vi "Edit Triton.vi"(8 "error in":errorcluster, 11 "Instrument parameters in":T1) -> (0 "error out":errorcluster, 3 "Instrument parameters (out)":T1)   [LabVIEW 2025]
uses:
  MyTriton.lvlib
panel:
  in  "Max Trial Number":i32
  in  "Select channel":u16(ring)=8 items=["PT2 Head"=1, "PT2 Plate"=2, "Still Plate"=3, "Cold Plate"=4, "MC Plate Cernox"=5, "PT1 Head"=6, "PT1 Plate"=7, "MC Plate RuO2"=8, "Magnet"=13]
  in  "Auto clear error?":bool=TRUE
  in  "Hold at end?":bool=TRUE
  in  "Initialize magnet?":bool
  in  "Precision":dbl=0.001
  in  "stop":bool
  # "Settings for Triton..."
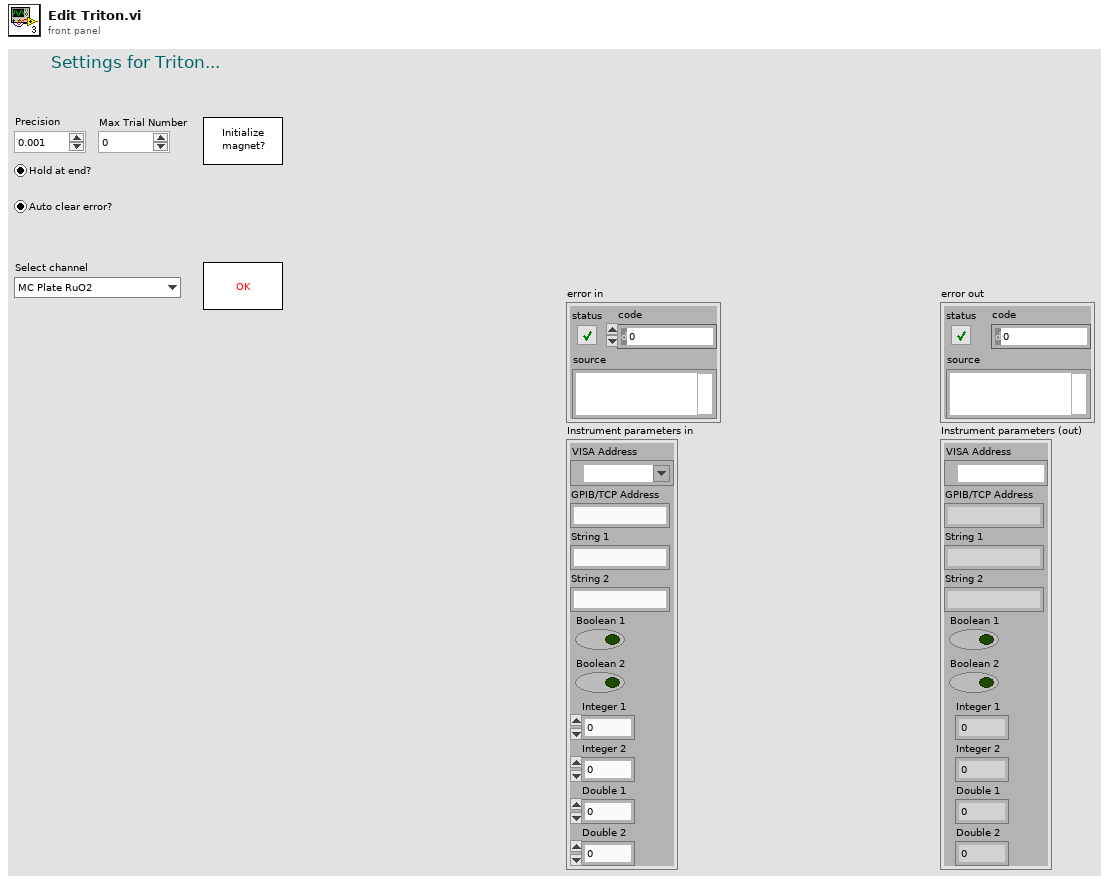
[diagram p1: front panel]
types:
  T1 = cluster{"VISA Address":refnum<visa-resource-name>, "GPIB/TCP Address":string, "String 1":string, "String 2":string, "Boolean 1":bool, "Boolean 2":bool, "Integer 1":i32, "Integer 2":i32, "Double 1":dbl, "Double 2":dbl}
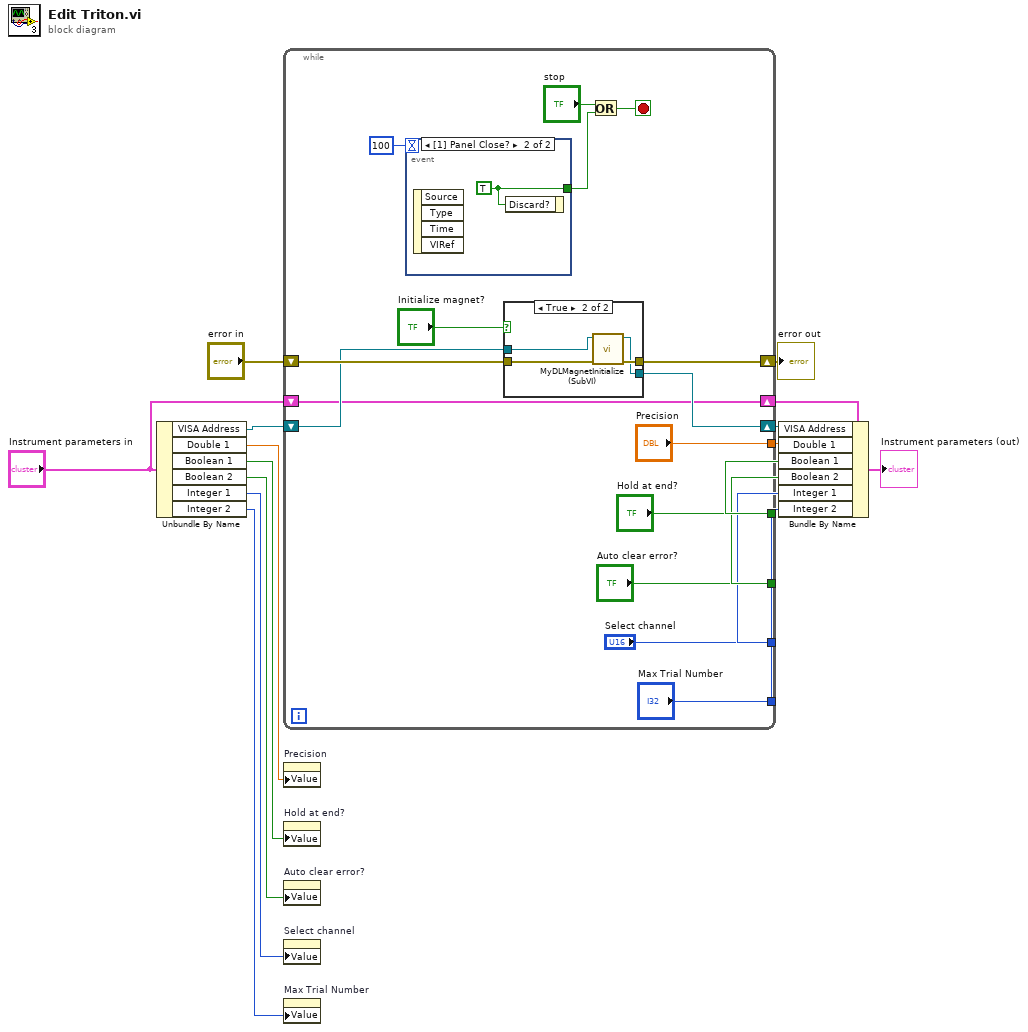
[diagram p0: block diagram]
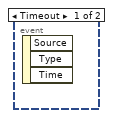
[diagram p3: hidden frame]
diagram:
  n1 = Unbundle By Name("Instrument parameters in") -> ("VISA Address"=w13:refnum<visa-resource-name>, "Double 1"=w14:dbl, "Boolean 1"=w5:bool, "Boolean 2"=w4:bool, "Integer 1"=w3:i32, "Integer 2"=w1:i32)
  n2 = while {
    shift-right: [w26] -> w16
    shift-left: "error in" -> [w27]
    shift-right: [w23] -> w11
    shift-left: "Instrument parameters in" -> [w23]
    shift-right: [w24] -> w10
    shift-left: w13 -> [w25]
    tunnel: ["Precision"] -> w12
    tunnel: ["Hold at end?"] -> w8
    tunnel: ["Auto clear error?"] -> w7
    tunnel: ["Select channel"] -> w6
    tunnel: ["Max Trial Number"] -> w2
    stop <- w29 stop-if-true
    n3 = event shown="[1] Panel Close?" {
      selector: _ -> [_ _]
      dyn-events: _ -> [_ _]
      timeout: 100 -> [_ _]
      tunnel: [_ w39] -> w30
      event Timeout {
        n4 = event-data() -> ()  [unwired: 1 in, 3 out]
      }
      event Panel Close? {
        w39 = TRUE ("Discard?")
        n5 = event-data() -> ()  [unwired: 1 in, 4 out]
        n6 = event-data("Discard?"=w39) -> ()  [unwired: 1 in, 1 out]
      }
    }
    n7 = case shown="True" "Initialize magnet?" {
      tunnel: w25 -> [w33 w38]
      tunnel: w27 -> [w34 w37]
      tunnel: [w34 w36] -> w26
      tunnel: [w33 w35] -> w24
      frame False {
      }
      frame True {
        n8 = call "MyDLMagnetInitialize (SubVI).vi"("error in"=w37, "VISA resource name in"=w38) -> ("error out"=w36:errorcluster, "VISA Refnum out"=w35:refnum<visa-resource-name>)  [unwired: 8 in]
      }
    }
    n9 = Or(x="stop", y=w30) -> (x .or. y?=w29:bool)
  }
  "error out" <- w16
  n10 = property on="Precision" class="DigNum (strict)"("Value"=w14) -> ()  [unwired: 2 in, 2 out]
  n11 = property on="Hold at end?" class="Bool (strict)"("Value"=w5) -> ()  [unwired: 2 in, 2 out]
  n12 = property on="Auto clear error?" class="Bool (strict)"("Value"=w4) -> ()  [unwired: 2 in, 2 out]
  n13 = property on="Select channel" class="Ring (strict)"("Value"=w3) -> ()  [unwired: 2 in, 2 out]
  n14 = property on="Max Trial Number" class="DigNum (strict)"("Value"=w1) -> ()  [unwired: 2 in, 2 out]
  n15 = Bundle By Name(cluster=w11, "VISA Address"=w10, "Double 1"=w12, "Boolean 1"=w8, "Boolean 2"=w7, "Integer 1"=w6, "Integer 2"=w2) -> (→"Instrument parameters (out)":T1)
